vi "UDP UI.vi"() -> ()   [LabVIEW 2015, in "E2E Tag Exchange editor node.lvclass"]
uses:
  E2E Tag Exchange editor node.lvclass
  object references.ctl
  <vilib>/NI/DCAF/Tag Editor Core/Configuration Editor/Classes/Engine Parent/Engine Parent Editor Node.lvclass
  references.ctl
  <vilib>/NI/Configuration Framework/Node/StopEvent.ctl
  <vilib>/NI/Configuration Framework/Node/RefreshUIEvent.ctl
  <vilib>/NI/Configuration Framework/Node/CacheState.ctl
  <vilib>/NI/Configuration Framework/Node/NodeChangeEvent.ctl
  <vilib>/NI/Configuration Framework/Node/NodeRef.ctl
  <vilib>/NI/Configuration Framework/Node/NISE_CEF_Node.lvclass
  <vilib>/NI/AMC/Message Queue.ctl
  <vilib>/NI/AMC/Message.ctl
  <vilib>/NI/Tools/Keyed Array/KeyedArray.ctl
  UDP UI References.ctl
  <vilib>/NI/Tools/Keyed Array/Tools_KeyedArray.lvlib
  <vilib>/NI/AMC/AMC.lvlib
panel:
  in  "References":T1
  in  "node References":T7
  out "Output Packet Size (bytes)":i32
  out "Input Packet Size (bytes)":i32
  in  "Tag":string(combo)
  in  "Generate":bool
  in  "Last Update Tag?":bool
  out "local_Address":string="localhost" caption="Address"
  in  "input_Local Port":u16 caption="Local Port (read from)"
  in  "Remote Port":u16 caption="Remote Port (write to)"
  in  "output_Local Port":u16 caption="Local Port (write from)"
  in  "Address":string
  # "Output"
  # "Input"
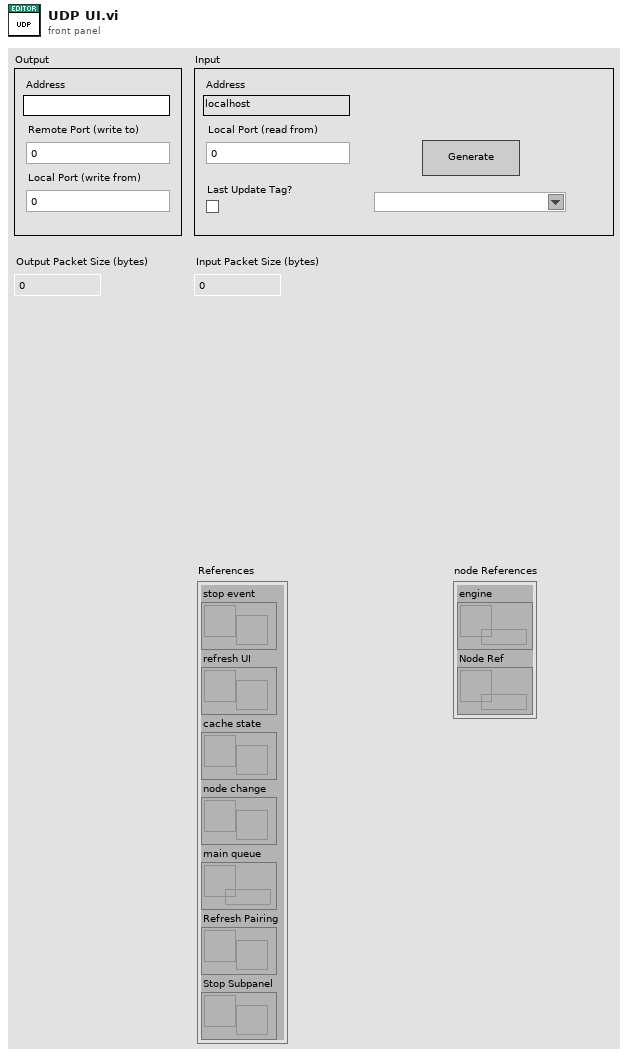
[diagram p1: front panel]
types:
  T1 = typedef "E2E Tag Exchange editor node.lvclass/references.ctl" = cluster{"stop event":T2, "refresh UI":T3, "cache state":T4, "node change":T5, "main queue":T6, "Refresh Pairing":refnum<user-event>, "Stop Subpanel":refnum<user-event>}
  T2 = typedef "NISE_CEF_Node.lvclass/StopEvent.ctl" = refnum<user-event>
  T3 = typedef "NISE_CEF_Node.lvclass/RefreshUIEvent.ctl" = refnum<user-event>
  T4 = typedef "NISE_CEF_Node.lvclass/CacheState.ctl" = refnum<user-event>
  T5 = typedef "NISE_CEF_Node.lvclass/NodeChangeEvent.ctl" = refnum<user-event>
  T6 = typedef "AMC.lvlib/Message Queue.ctl" = refnum<queue>
  T7 = typedef "E2E Tag Exchange editor node.lvclass/object references.ctl" = cluster{"engine":refnum<data-value>, "Node Ref":refnum<data-value>}
  T8 = typedef "E2E Tag Exchange editor node.lvclass/UDP UI References.ctl" = cluster{"Address":refnum<vi>, "Remote Port":refnum<vi>, "input_Local Port":refnum<vi>, "output_Local Port":refnum<vi>, "Last Update Tag?":refnum<vi>, "Tag":refnum<vi>, "Generate":refnum<vi>, "Input Packet Size":refnum<vi>, "Output Packet Size":refnum<vi>}
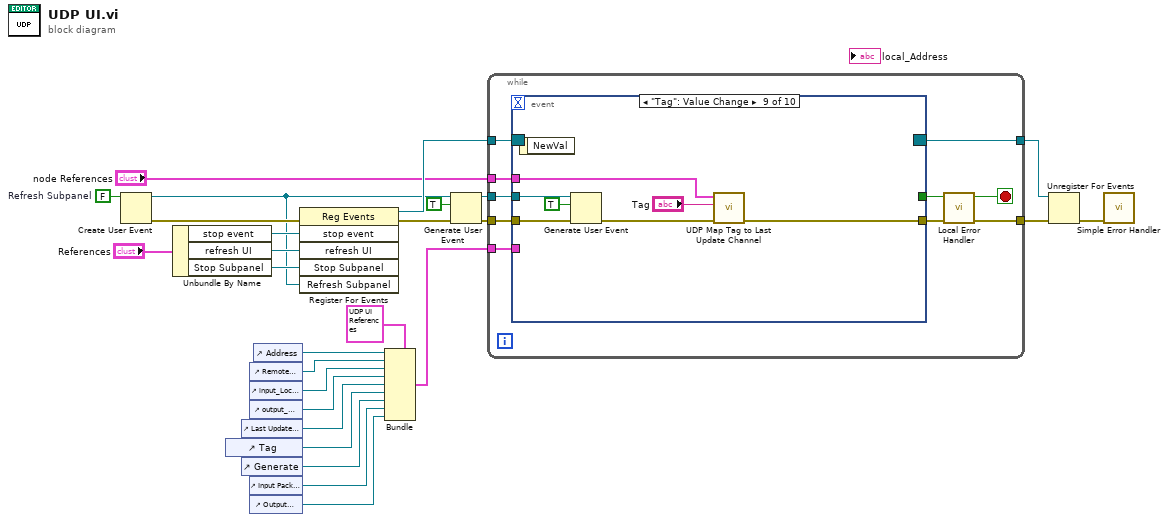
[diagram p0: block diagram]
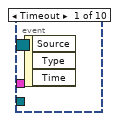
[diagram p2: hidden frame]
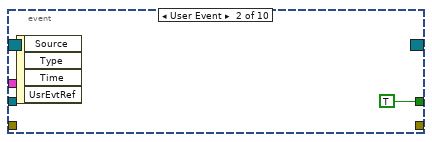
[diagram p3: hidden frame]
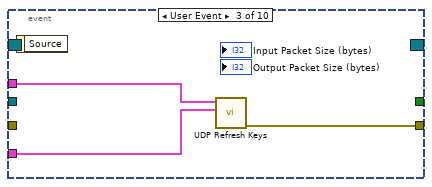
[diagram p4: hidden frame]
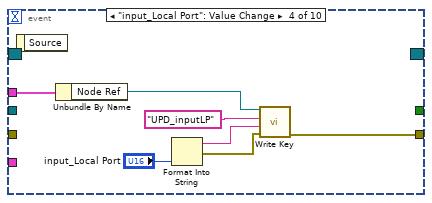
[diagram p5: hidden frame]
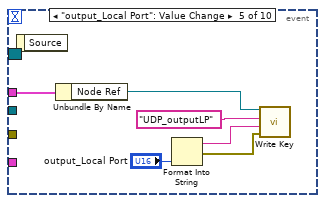
[diagram p6: hidden frame]
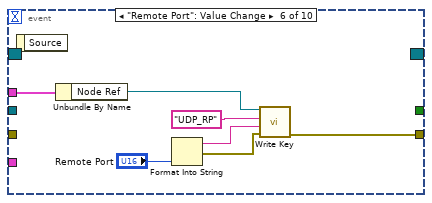
[diagram p7: hidden frame]
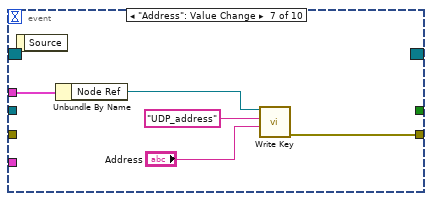
[diagram p8: hidden frame]
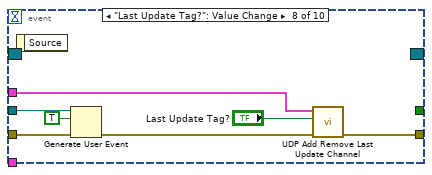
[diagram p9: hidden frame]
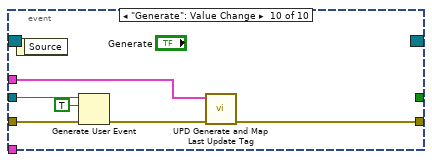
[diagram p10: hidden frame]
diagram:
  w21 = FALSE  # Refresh Subpanel
  n1 = Create User Event(user event datatype=w21) -> (user event=w1:refnum<user-event>, error out=w5:errorcluster)  [unwired: 1 in]
  n2 = Unbundle By Name("References") -> ("stop event"=w26:T2, "refresh UI"=w25:T3, "Stop Subpanel"=w24:refnum<user-event>)
  n3 = control-ref of="Tag"() -> (w14:refnum<vi>)
  n4 = control-ref of="Last Update Tag?"() -> (w15:refnum<vi>)
  n5 = control-ref of="Generate"() -> (w13:refnum<vi>)
  n6 = control-ref of="Remote Port"() -> (w18:refnum<vi>)
  n7 = control-ref of="input_Local Port"() -> (w17:refnum<vi>)
  n8 = control-ref of="output_Local Port"() -> (w16:refnum<vi>)
  n9 = control-ref of="Input Packet Size (bytes)"() -> (w11:refnum<vi>)
  n10 = control-ref of="Output Packet Size (bytes)"() -> (w10:refnum<vi>)
  n11 = control-ref of="Address"() -> (w19:refnum<vi>)
  n12 = register-events(error in=w5, w26, w25, w24, w1) -> (reference out=w23:refnum<event-registration>, error out=w4:errorcluster)  [unwired: 1 in]
  n13 = Bundle(cluster=T8 {"Address"=refnum, "Remote Port"=refnum, "input_Local Port"=refnum, "output_Local Port"=refnum, "Last Update Tag?"=refnum, "Tag"=refnum, "Generate"=refnum, "Input Packet Size"=refnum, "Output Packet Size"=refnum} ("UDP UI References"), "Address"=w19, "Remote Port"=w18, "input_Local Port"=w17, "output_Local Port"=w16, "Last Update Tag?"=w15, "Tag"=w14, "Generate"=w13, "Input Packet Size"=w11, "Output Packet Size"=w10) -> (w12:T8)
  n14 = Generate User Event(user event=w1, event data cluster=TRUE ("event data"), error in=w4) -> (user event out=w2:refnum<user-event>, error out=w3:errorcluster)  [unwired: 1 in]
  n15 = while {
    tunnel: w23 -> [w37]
    tunnel: w3 -> [w36]
    tunnel: "node References" -> [w35]
    tunnel: w2 -> [w34]
    tunnel: w12 -> [w33]
    tunnel: [w29] -> w8
    tunnel: [w28] -> w7
    stop <- w31 stop-if-true
    n16 = event shown="[8] \"Tag\": Value Change" {
      selector: w37 -> [_ _ _ _ _ _ _ _ _ _]
      dyn-events: [_ _ _ _ _ _ _ _ _ _] -> w29
      timeout: _ -> [_ _ _ _ _ _ _ _ _ _]
      tunnel: w36 -> [_ _ _ _ _ _ _ w68 w76 w82]
      tunnel: [_ TRUE _ _ _ _ _ _ _ _] -> w30
      tunnel: w35 -> [_ _ w39 w48 w54 w61 w66 w72 w79 w86]
      tunnel: [_ _ w41 w42 _ w55 w63 w73 w80 w85] -> w32
      tunnel: w34 -> [_ _ _ _ _ _ _ w69 w75 w83]
      tunnel: w33 -> [_ _ w40 _ _ _ _ _ _ _]
      event Timeout {
        n17 = event-data() -> ()  [unwired: 1 in, 3 out]
      }
      event User Event {
        n18 = event-data() -> ()  [unwired: 1 in, 4 out]
      }
      event User Event {
        n19 = event-data() -> ()  [unwired: 1 in, 1 out]
        n20 = call "UDP Refresh Keys.vi"("UDP UI References"=w40, "node References"=w39) -> ("error out"=w41:errorcluster)  [unwired: 7 in, 2 out]
      }
      event "input_Local Port": Value Change {
        n21 = event-data() -> ()  [unwired: 1 in, 1 out]
        n22 = Unbundle By Name(w48) -> ("Node Ref"=w47:refnum<data-value>)
        n23 = Format Into String("input_Local Port") -> (resulting string=w45:string, error out=w44:errorcluster)  [unwired: 3 in]
        n24 = call "Write Key.vi"("error in (no error)"=w44, "Value"=w45, "Key"="UPD_inputLP", "E2E editor node in"=w47) -> ("error out"=w42:errorcluster)  [unwired: 6 in, 1 out]
      }
      event "output_Local Port": Value Change {
        n25 = event-data() -> ()  [unwired: 1 in, 1 out]
        n26 = Unbundle By Name(w54) -> ("Node Ref"=w53:refnum<data-value>)
        n27 = Format Into String("output_Local Port") -> (resulting string=w52:string, error out=w51:errorcluster)  [unwired: 3 in]
        n28 = call "Write Key.vi"("error in (no error)"=w51, "Value"=w52, "Key"="UDP_outputLP", "E2E editor node in"=w53) -> ()  [unwired: 6 in, 2 out]
      }
      event "Remote Port": Value Change {
        n29 = event-data() -> ()  [unwired: 1 in, 1 out]
        n30 = Unbundle By Name(w61) -> ("Node Ref"=w60:refnum<data-value>)
        n31 = Format Into String("Remote Port") -> (resulting string=w59:string, error out=w58:errorcluster)  [unwired: 3 in]
        n32 = call "Write Key.vi"("error in (no error)"=w58, "Value"=w59, "Key"="UDP_RP", "E2E editor node in"=w60) -> ("error out"=w55:errorcluster)  [unwired: 6 in, 1 out]
      }
      event "Address": Value Change {
        n33 = event-data() -> ()  [unwired: 1 in, 1 out]
        n34 = Unbundle By Name(w66) -> ("Node Ref"=w65:refnum<data-value>)
        n35 = call "Write Key.vi"("Value"="Address", "Key"="UDP_address", "E2E editor node in"=w65) -> ("error out"=w63:errorcluster)  [unwired: 7 in, 1 out]
      }
      event "Last Update Tag?": Value Change {
        n36 = event-data() -> ()  [unwired: 1 in, 1 out]
        n37 = Generate User Event(user event=w69, event data cluster=TRUE, error in=w68) -> (error out=w67:errorcluster)  [unwired: 1 in, 1 out]
        n38 = call "UDP Add Remove Last Update Channel.vi"("error in (no error)"=w67, "Last Update Tag?"="Last Update Tag?", "node References"=w72) -> ("error out"=w73:errorcluster)  [unwired: 7 in, 1 out]
      }
      event "Tag": Value Change {
        n39 = event-data() -> ()  [unwired: 1 in, 1 out]
        n40 = Generate User Event(user event=w75, event data cluster=TRUE, error in=w76) -> (error out=w74:errorcluster)  [unwired: 1 in, 1 out]
        n41 = call "UDP Map Tag to Last Update Channel.vi"("error in (no error)"=w74, "Tag Name"="Tag", "node References"=w79) -> ("error out"=w80:errorcluster)  [unwired: 7 in, 1 out]
      }
      event "Generate": Value Change {
        n42 = event-data() -> ()  [unwired: 1 in, 1 out]
        n43 = Generate User Event(user event=w83, event data cluster=TRUE ("event data"), error in=w82) -> (error out=w81:errorcluster)  [unwired: 1 in, 1 out]
        n44 = call "UPD Generate and Map Last Update Tag.vi"("error in (no error)"=w81, "node References"=w86) -> ("error out"=w85:errorcluster)  [unwired: 8 in, 1 out]
      }
    }
    n45 = call "Local Error Handler.vi"("error in"=w32, "Stop in"=w30) -> ("error out"=w28:errorcluster, "Stop out"=w31:bool)  [unwired: 8 in]
  }
  n46 = Unregister For Events(event registration refnum=w8, error in=w7) -> (error out=w6:errorcluster)
  n47 = call <vilib>:"Simple Error Handler.vi"("error in (no error)"=w6) -> ()  [unwired: 4 in, 5 out]
